vi "New Run Object.vi"(7 "xwpfRun Type":refnum<class "xwpfRun.lvclass">, 8 "error in (no error)":errorcluster, 11 "Run Ref":refnum<k24>) -> (0 "error out":errorcluster, 3 "xwpfRun out":refnum<class "xwpfRun.lvclass">)   [LabVIEW 2017, in "Word_Specific.lvlib" / "xwpfRun.lvclass"]
uses:
  xwpfRun.lvclass
  C:/Users/Neo/Desktop/Dev_Tools_BR/LabVIEW_NPOI/src/lib/NPOI 2.1.1/NPOI.OOXML.dll
  lib/NPOI 2.1.1/NPOI.OOXML.dll
  xwpfRun.lvclass/xwpfRun.ctl
  Set Run Ref.vi
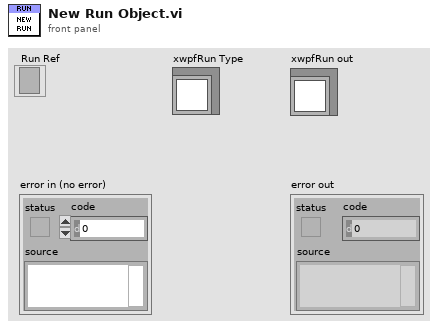
[diagram p1: front panel]
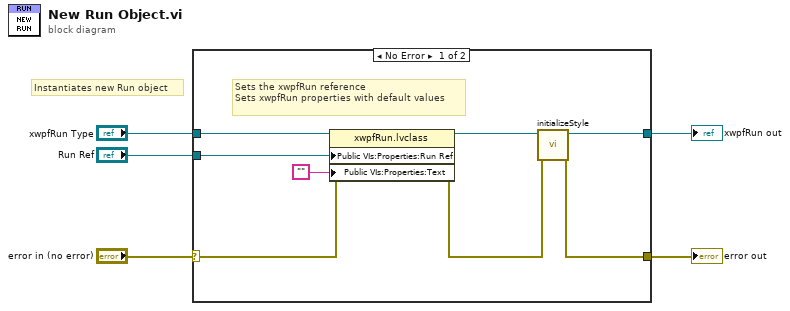
[diagram p0: block diagram]
diagram:
  # "Instantiates new Run object"
  n1 = case shown="No Error" "error in (no error)" {
    selector: "error in (no error)" -> [w9 w15]
    tunnel: [w6 w15] -> w4
    tunnel: [w8 w14] -> w2
    tunnel: "xwpfRun Type" -> [w13 w14]
    tunnel: "Run Ref" -> [w11 _]
    frame No Error {
      # "Sets the xwpfRun reference\nSets xwpfRun properties with default values"
      n2 = property class="xwpfRun.lvclass"(reference=w13, error in=w9, "Public VIs:Properties:Run Ref"=w11, "Public VIs:Properties:Text"="") -> (reference out=w12:refnum<class "xwpfRun.lvclass">, error out=w7:errorcluster)
      n3 = call-dynamic "initializeStyle.vi"("error in (no error)"=w7, "xwpfRun in"=w12) -> ("error out"=w6:errorcluster, "xwpfRun out"=w8:refnum<class "xwpfRun.lvclass">)  [unwired: 8 in]
    }
    frame Error {
    }
  }
  "error out" <- w4
  "xwpfRun out" <- w2
